vi "VALEW_LE_Knob Select (SLB).vi"(0 "Knob":enum16{"One", "Two", "Three", "Four"}(ring), 5 "Knob Position":i32(ring) items=["Invalid"=6, "Six"=5, "Five"=4, "Four"=3, "Three"=2, "Two"=1, "One"=0], 7 "Number of positions":i32(ring)=2 items=["Six"=5, "Five"=4, "Four"=3, "Three"=2], 11 "Error In":errorcluster) -> (15 "Error Out":errorcluster)   [LabVIEW 2016, in "2015 VA Washer.lvlib"]
uses:
  Projects/2015 VA Washer.lvlib
  <vilib>/DAQmx/write.llb/DAQmx Write (Analog DBL 1Chan 1Samp).vi
  <vilib>/DAQmx/create/channels.llb/DAQmx Create Channel (AO-Voltage-Basic).vi
  <vilib>/DAQmx/miscellaneous.llb/DAQmx Fill In Error Info.vi
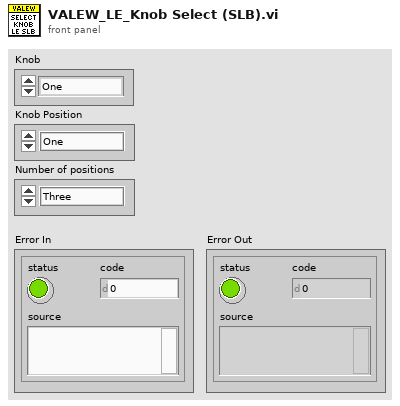
[diagram p1: front panel]
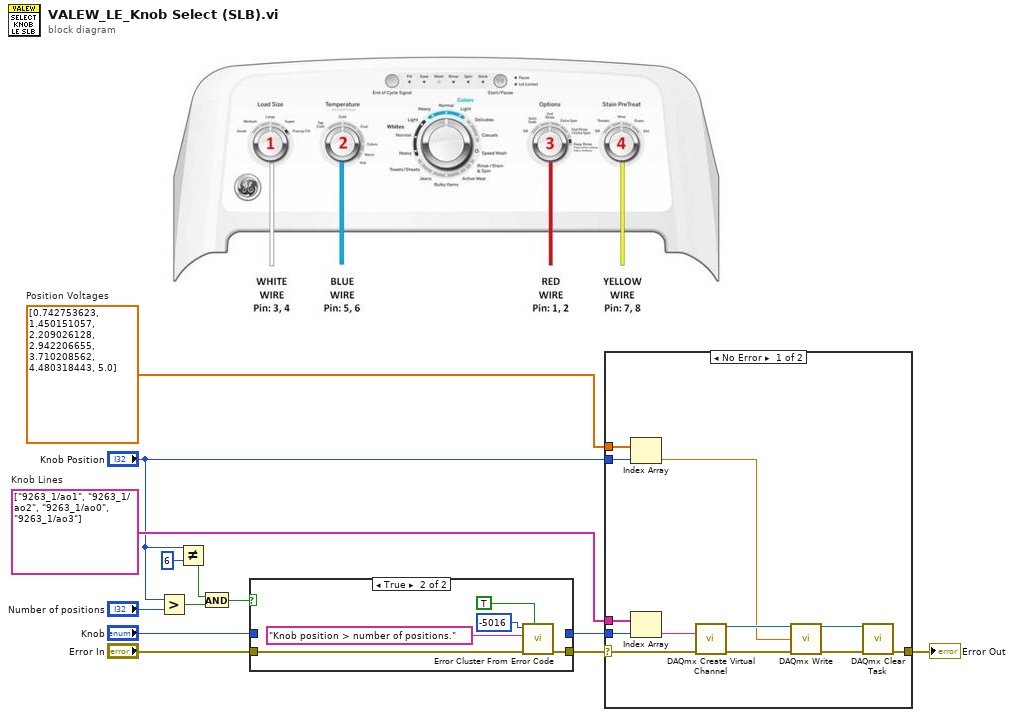
[diagram p0: block diagram]
diagram:
  w12 = tag[] ["9263_1/ao1", "9263_1/ao2", "9263_1/ao0", "9263_1/ao3"]  # Knob Lines
  w11 = dbl[] [0.742753623, 1.450151057, 2.209026128, 2.942206655, 3.710208562, 4.480318443, 5.0]  # Position Voltages
  n1 = Greater?(x="Knob Position", y="Number of positions") -> (0:w2:bool)
  n2 = Not Equal?(x="Knob Position", y=6) -> (x != y?=w3:bool)
  n3 = And(x=w3, y=w2) -> (x .and. y?=w1:bool)
  n4 = case shown="True" w1 {
    tunnel: [w15 w17] -> w9
    tunnel: "Error In" -> [w15 w16]
    tunnel: [w14 _] -> w7
    tunnel: "Knob" -> [w14 _]
    frame False {
    }
    frame True {
      n5 = call <vilib>:"Error Cluster From Error Code.vi"("show call chain? (False)"=TRUE, "error in (no error)"=w16, "error message (\"\")"="Knob position > number of positions." ("error message (\"\")"), "error code (0)"=-5016) -> ("error out"=w17:errorcluster)  [unwired: 5 in]
    }
  }
  n6 = case shown="No Error" w9 {
    selector: w9 -> [w24 w33]
    tunnel: "Knob Position" -> [w27 _]
    tunnel: w7 -> [w32 _]
    tunnel: w12 -> [w31 _]
    tunnel: w11 -> [w26 _]
    tunnel: [w21 w33] -> w10
    frame No Error {
      n7 = Index Array(array=w26, index=w27) -> (element=w25:dbl)
      n8 = Index Array(array=w31, index=w32) -> (element=w30:tag)
      n9 = call-poly <vilib>:"DAQmx Create Virtual Channel.vi"("physical channels"=w30, "error in"=w24) -> ("task out"=w29:refnum<k21>, "error out"=w28:errorcluster)  [unwired: 12 in]
      n10 = call-poly <vilib>:"DAQmx Write.vi"("task/channels in"=w29, "data"=w25, "error in"=w28) -> ("task out"=w23:refnum<k21>, "error out"=w22:errorcluster)  [unwired: 10 in, 1 out]
      n11 = call <vilib>:"DAQmx Clear Task.vi"("task in"=w23, "error in"=w22) -> ("error out"=w21:errorcluster)  [unwired: 13 in]
    }
    frame Error {
    }
  }
  "Error Out" <- w10
